vi "Send Command.vi"(8 "error in (no error)":errorcluster, 10 "write buffer":string, 11 "VISA resource name In":refnum<visa-resource-name>) -> (0 "error out":errorcluster, 3 "VISA resource name out":refnum<visa-resource-name>)   [LabVIEW 2013, in "Newport 1830-C.lvlib"]
doc: "Sends a command using the VISA drivers then waits sepecified ms."
uses:
  Newport 1830-C.lvlib
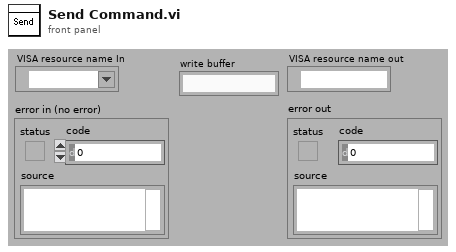
[diagram p1: front panel]
types:
  T1 = typedef "Semaphore RefNum" = refnum<k1>
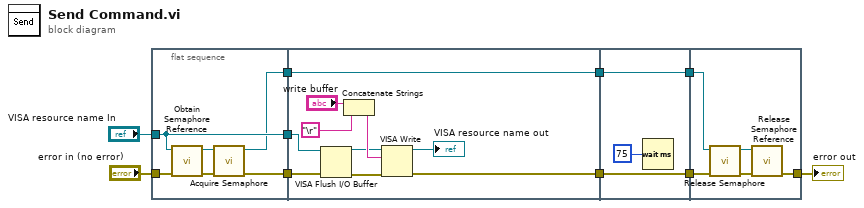
[diagram p0: block diagram]
diagram:
  n1 = flat-sequence {
    tunnel: "VISA resource name In" -> [w12]
    tunnel: [w12] -> w6
    tunnel: [w14] -> w5
    tunnel: "error in (no error)" -> [w13]
    tunnel: [w11] -> w3
    tunnel: [w25] -> w8
    tunnel: w6 -> [w20]
    tunnel: w5 -> [w21]
    tunnel: w3 -> [w17]
    tunnel: [w17] -> w1
    tunnel: [w29] -> w9
    tunnel: w8 -> [w29]
    tunnel: [w27] -> w2
    tunnel: w1 -> [w27]
    tunnel: w9 -> [w34]
    tunnel: [w31] -> w7
    tunnel: w2 -> [w30]
    frame #0 {
      n2 = call <vilib>:"Obtain Semaphore Reference.vi"("error in (no error)"=w13, "name (unnamed)"=w12) -> ("error out"=w15:errorcluster, "semaphore"=w16:T1)  [unwired: 3 in, 1 out]
      n3 = call <vilib>:"Acquire Semaphore.vi"("error in (no error)"=w15, "semaphore"=w16) -> ("error out"=w14:errorcluster, "semaphore out"=w11:T1)  [unwired: 3 in, 1 out]
    }
    frame #1 {
      n4 = VISA Flush I/O Buffer(VISA resource name=w20, error in (no error)=w21) -> (VISA resource name out=w18:refnum<visa-resource-name>, error out=w19:errorcluster)  [unwired: 1 in]
      n5 = Concatenate Strings("write buffer", "\r") -> (w22:string)
      n6 = VISA Write(VISA resource name=w18, write buffer=w22, error in (no error)=w19) -> (VISA resource name out=→"VISA resource name out":refnum<visa-resource-name>, error out=w25:errorcluster)  [unwired: 1 out]
    }
    frame #2 {
      n7 = Wait (ms)(milliseconds to wait=u32 75) -> ()  [unwired: 1 out]
    }
    frame #3 {
      n8 = call <vilib>:"Release Semaphore.vi"("error in (no error)"=w34, "semaphore"=w30) -> ("error out"=w33:errorcluster, "semaphore out"=w32:T1)  [unwired: 4 in]
      n9 = call <vilib>:"Release Semaphore Reference.vi"("error in (no error)"=w33, "semaphore"=w32) -> ("error out"=w31:errorcluster)  [unwired: 8 in, 1 out]
    }
  }
  "error out" <- w7
